vi "Align with Target Implementation.vi"(8 "Deadband (°)":dbl) -> (0 "Finished?":bool, 3 "Power Setpoint":dbl)   [LabVIEW 2019]
uses:
  Framework/Robot Global Data.vi
  Turret Published Globals.vi
  <vilib>/addons/control/pid/pid.llb/PID (DBL).vi
  <vilib>/addons/control/pid/NI_PID_pid.lvlib
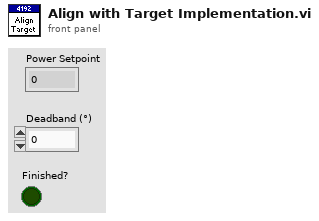
[diagram p1: front panel]
types:
  T1 = cluster{"Shooter Velocity":cluster{"Sensor Velocity":dbl, "Setpoint":dbl, "Applied Output":dbl}, "Turret Position":cluster{"output":dbl, "Horizontal Offset":dbl}, "Hood Position":cluster{"Sensor Velocity":dbl, "Setpoint":dbl, "Applied Output":dbl}, "Shooter PID Constants":cluster{"P Gain":dbl, "I Gain":dbl, "D Gain":dbl, "F Gain":dbl, "I Zone":dbl, "Min Output":dbl, "Max Output":dbl}, "Hood PID Constants":cluster{"P Gain":dbl, "I Gain":dbl, "D Gain":dbl, "F Gain":dbl, "I Zone":dbl, "Min Output":dbl, "Max Output":dbl}, "Turret PID Constants":cluster{"P Gain":dbl, "I Gain":dbl, "D Gain":dbl, "F Gain":dbl, "I Zone":dbl, "Min Output":dbl, "Max Output":dbl}, "Limelight PID Gains":cluster{"proportional gain (Kc)":dbl, "integral time (Ti, min)":dbl, "derivative time (Td, min)":dbl}}
  T2 = cluster{"Valid Target":bool, "Horizontal Offset":dbl, "Vertical Offset":dbl, "Target Area":dbl, "Skew":dbl}
  T3 = cluster{"proportional gain (Kc)":dbl, "integral time (Ti, min)":dbl, "derivative time (Td, min)":dbl}
  T4 = cluster{"Shooter Up To Speed?":bool, "Aligned With Target?":bool, "Hood at Angle?":bool, "Shooting?":bool, "Hood Angle":dbl, "Turret Angle":dbl}
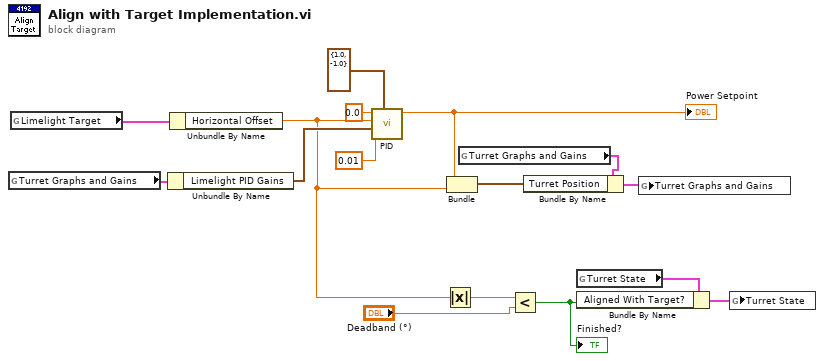
[diagram p0: block diagram]
diagram:
  n1 = global read "Turret Published Globals.vi" "Turret Graphs and Gains"() -> (w13:T1)
  n2 = global read "Robot Global Data.vi" "Limelight Target"() -> (w6:T2)
  n3 = Unbundle By Name(w13) -> ("Limelight PID Gains"=w14:T3)
  n4 = Unbundle By Name(w6) -> ("Horizontal Offset"=w12:dbl)
  n5 = call-poly <vilib>:"PID.vi"("output range"=cluster{"output high":dbl, "output low":dbl} {"output high"=1.0, "output low"=-1.0}, "dt (s)"=0.01, "PID gains"=w14, "process variable"=w12, "setpoint"=0.0) -> ("output"=w11:dbl)  [unwired: 5 in, 1 out]
  "Power Setpoint" <- w11
  n6 = Absolute Value(x=w12) -> (abs(x)=w10:dbl)
  n7 = Bundle("output"=w11, "Horizontal Offset"=w12) -> (w3:cluster{"output":dbl, "Horizontal Offset":dbl})  [unwired: 1 in]
  n8 = global read "Turret Published Globals.vi" "Turret Graphs and Gains"() -> (w2:T1)
  n9 = Less?(x=w10, y="Deadband (°)") -> (x < y?=w4:bool)
  "Finished?" <- w4
  n10 = Bundle By Name(cluster=w2, "Turret Position"=w3) -> (w1:T1)
  n11 = global read "Turret Published Globals.vi" "Turret State"() -> (w15:T4)
  n12 = Bundle By Name(cluster=w15, "Aligned With Target?"=w4) -> (w16:T4)
  n13 = global write "Turret Published Globals.vi" "Turret Graphs and Gains"(w1) -> ()
  n14 = global write "Turret Published Globals.vi" "Turret State"(w16) -> ()
